vi "Simulate3DOFChair.vi"(0 "array":dbl[][](array[numeric])=[[80.0, 80.0]], 1 "L_seat":dbl=40.0, 2 "L_back":dbl=40.0, 5 "origin":cluster{"x":i16, "y":i16}, 7 "Reflection":cluster{"x":i16, "y":i16}={"x"=1, "y"=1}, 9 "L1":dbl=80.0, 11 "L2":dbl=80.0, 12 "Empty picture":picture) -> (4 "2D Picture 2":picture, 6 "point to IK":cluster{dbl, dbl})   [LabVIEW 2024]
panel:
  out "theta3":dbl(knob)=-96.67737485561672 scale=-90.0..90.0
  out "end eff coords":cluster{"x2":dbl, "y2":dbl}={"x2"=70.00000000000001, "y2"=90.0}
  out "Arm 1 coords":cluster{"x":dbl, "y":dbl}={"x"=79.30228332368782, "y"=10.542668526020577}
  in  "Empty Array 2":dbl[][](array[numeric])
  out "Drawn Coords":dbl[][](array[numeric])=[[70.00000000000001, 90.0]]
  out "angle 2":dbl=52.125016348901795
  out "mag 2":dbl=114.01754250991381
  out "end effector":cluster{dbl, dbl}={70.00000000000001, 90.0} caption="end effector 2" {"?" format="%.1f"; "?" format="%#.1f"}
  out "theta 2":dbl(knob)=89.10471701342988 scale=-90.0..90.0
  out "theta 1":dbl(knob)=7.572657842186857 scale=-90.0..90.0
  # "mm"
  # "mm"
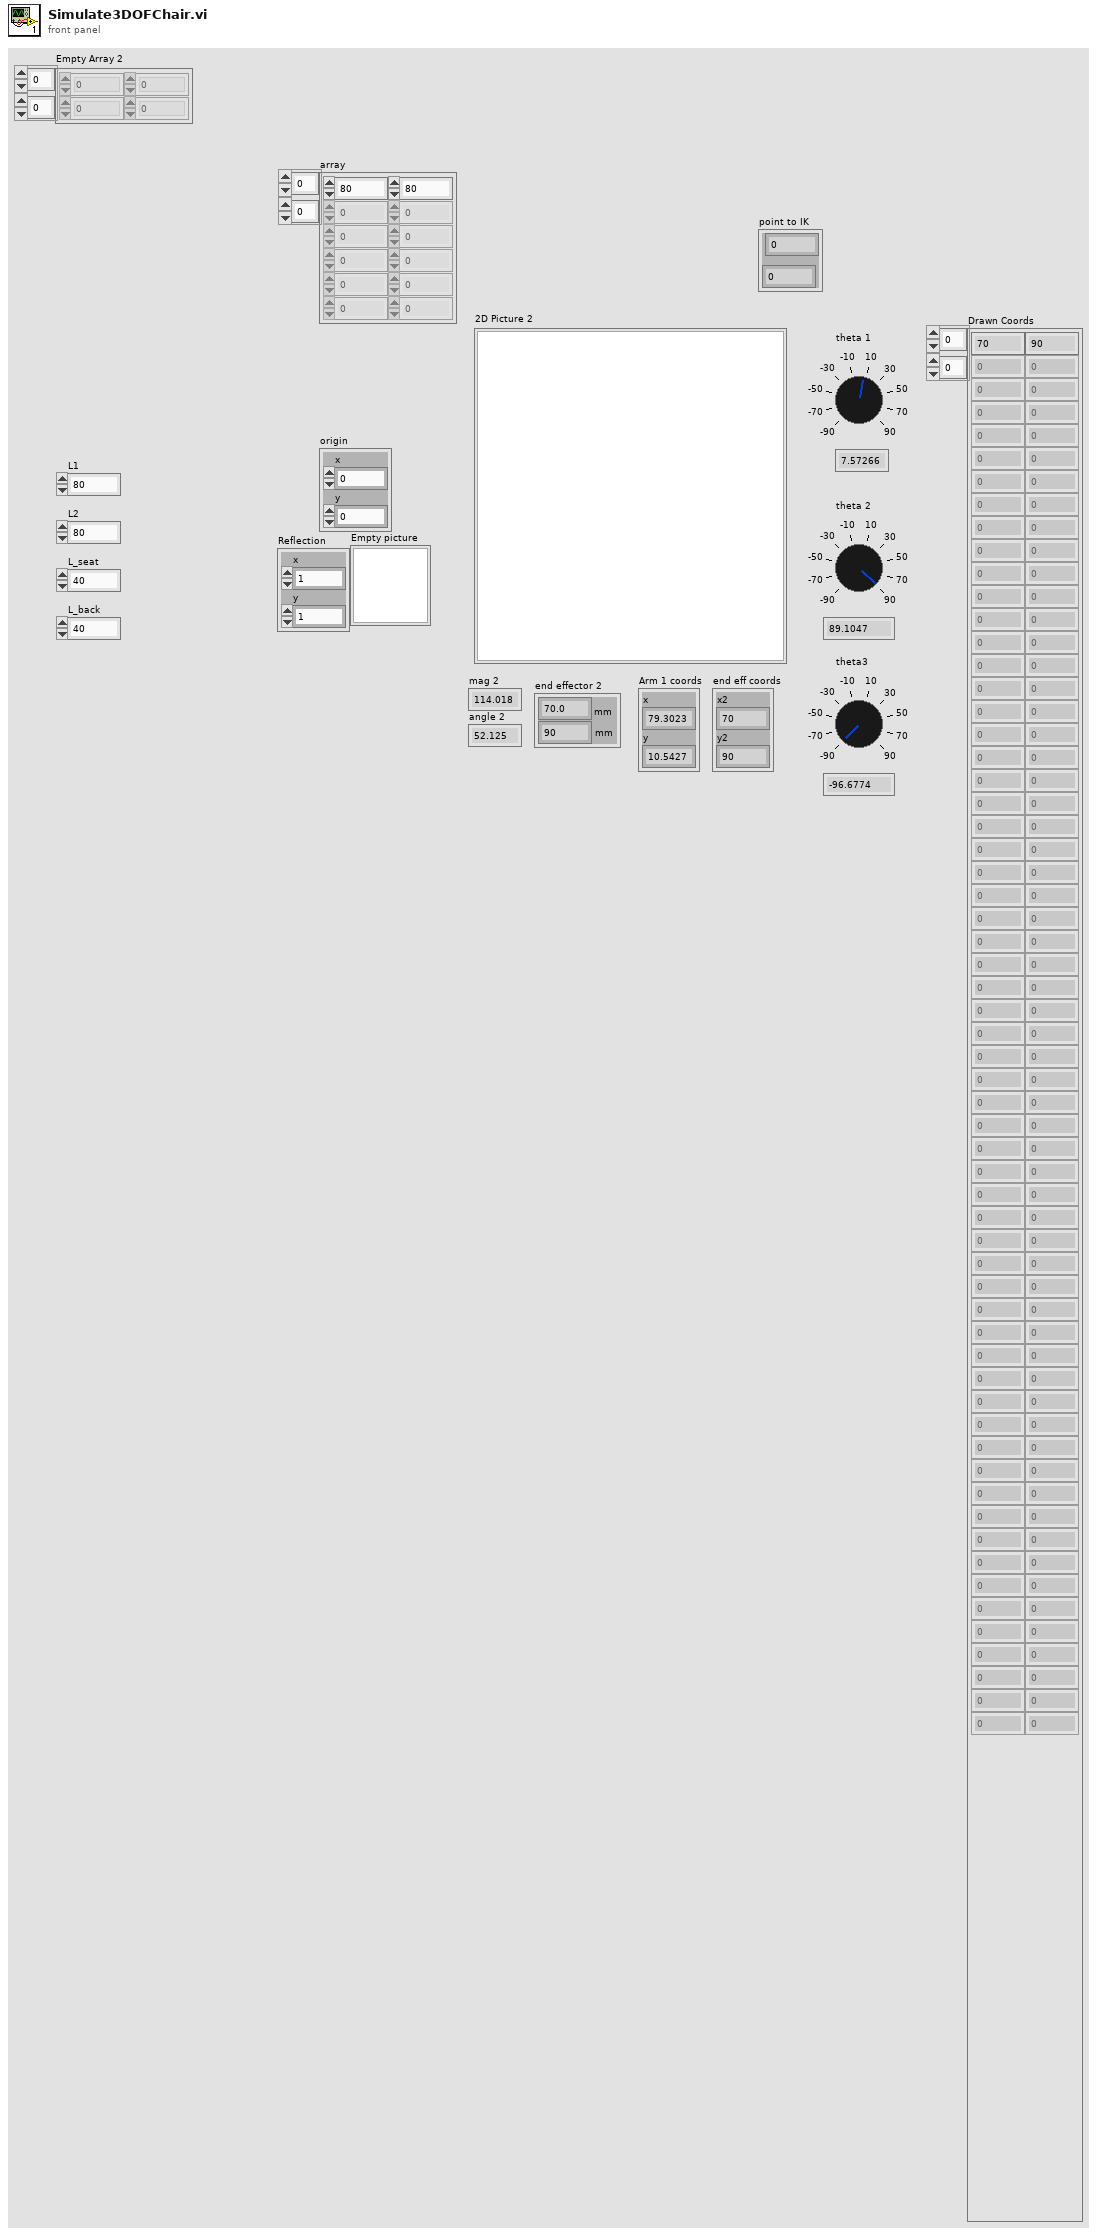
[diagram p1: front panel]
types:
  T1 = cluster{"Width":u16, "Style":enum32{"Solid", "Dash", "Dot", "DashDot", "DashDotDot"}}
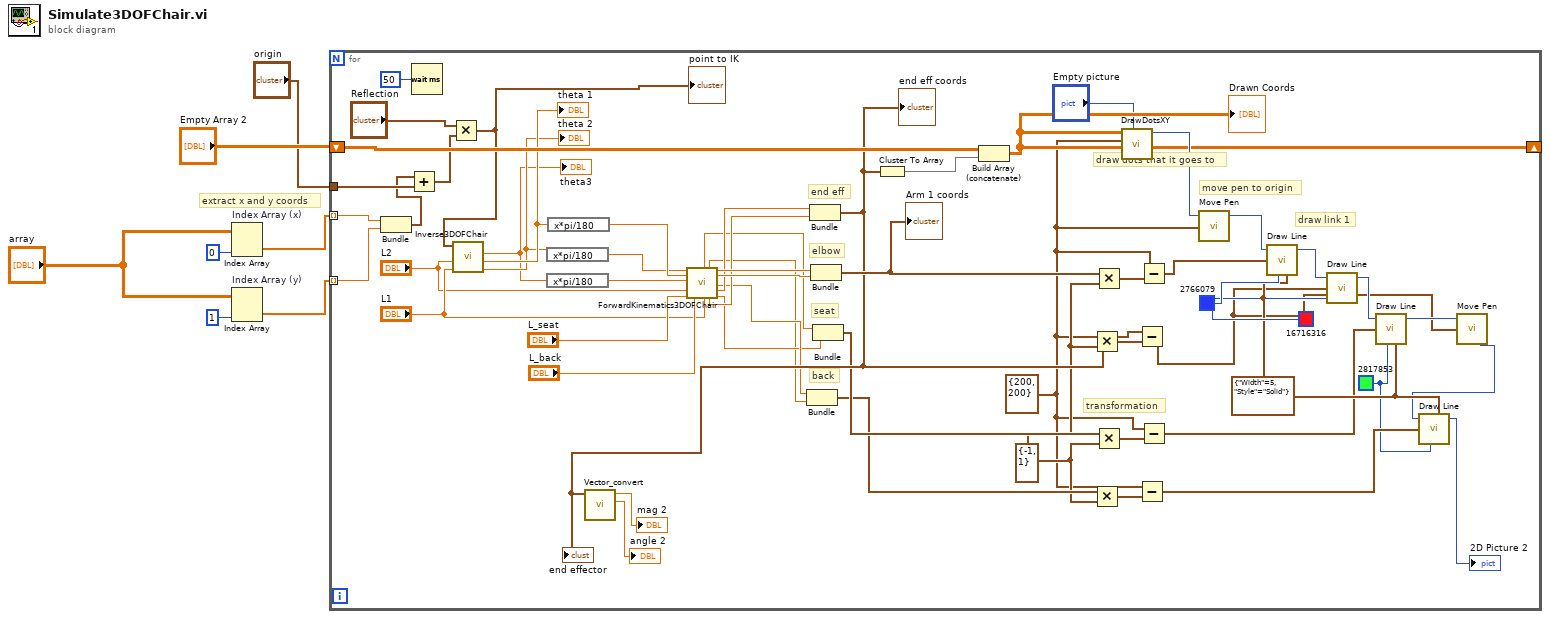
[diagram p0: block diagram]
diagram:
  # "extract x and y coords"
  n1 = Index Array "Index Array (x)"(array="array", index (col)=0 ("index (row)")) -> (element=w4:dbl[])  [unwired: 1 in]
  n2 = Index Array "Index Array (y)"(array="array", index (col)=1 ("index (row)")) -> (element=w5:dbl[])  [unwired: 1 in]
  n3 = for {
    tunnel: w4 -> [w50] mode=indexing
    tunnel: w5 -> [w49] mode=indexing
    shift-right: [w36] -> _
    shift-left: "Empty Array 2" -> [w58]
    tunnel: "origin" -> [w13]
    w24 = u32 2817853 ("color(black)")
    w27 = cluster{"x":i16, "y":i16} {"x"=-1, "y"=1} ("new position")
    w30 = T1 {"Width"=5, "Style"=enum."Solid"} ("pen")
    w26 = cluster{"x":i16, "y":i16} {"x"=200, "y"=200} ("new position")
    # "draw link 1"
    # "move pen to origin"
    # "draw dots that it goes to"
    # "back"
    # "seat"
    # "transformation"
    # "end eff"
    # "elbow"
    n4 = Bundle("y (mm)"=w50, "y (mm)"=w49) -> (w12:cluster{"y (mm)":dbl, "y (mm)":dbl})  [unwired: 1 in]
    n5 = Add(x=w12, y=w13) -> (x+y=w10:cluster{dbl, dbl})
    n6 = Wait (ms)(milliseconds to wait=u32 50) -> ()  [unwired: 1 out]
    n7 = Multiply(x="Reflection", y=w10) -> (x*y=w9:cluster{dbl, dbl})
    "point to IK" <- w9
    n8 = call "Inverse3DOFChair.vi"("L 2"="L1", "L 1"="L2", "end effector"=w9) -> ("theta2"=w17:dbl, "theta1"=w19:dbl, "theta3"=w15:dbl)  [unwired: 6 in]
    "theta 1" <- w19
    "theta 2" <- w17
    "theta3" <- w15
    n9 = expression code="x*pi/180"(w17) -> (w16:dbl)
    n10 = expression code="x*pi/180"(w15) -> (w14:dbl)
    n11 = expression code="x*pi/180"(w19) -> (w18:dbl)
    n12 = call "ForwardKinematics3DOFChair.vi"("theta2"=w16, "theta1"=w18, "L2"="L2", "seat"="L_seat", "theta3"=w14, "back"="L_back", "L1"="L1") -> ("x3"=w38:dbl, "y4"=w37:dbl, "y2"=w45:dbl, "x1"=w48:dbl, "y1"=w47:dbl, "x4"=w40:dbl, "x2"=w46:dbl, "y3"=w39:dbl)  [unwired: 5 in]
    n13 = Bundle("x4"=w40, "y4"=w37) -> (w28:cluster{"x4":dbl, "y4":dbl})  [unwired: 1 in]
    n14 = Bundle("x2"=w46, "y2"=w45) -> (w51:cluster{"x2":dbl, "y2":dbl})  [unwired: 1 in]
    "end effector" <- w51
    "end eff coords" <- w51
    n15 = call "Vector_convert.vi"("x,y"=w51) -> ("angle"=→"angle 2":dbl, "mag"=→"mag 2":dbl)  [unwired: 9 in]
    n16 = Bundle("x1"=w48, "y1"=w47) -> (w53:cluster{"x1":dbl, "y1":dbl})  [unwired: 1 in]
    "Arm 1 coords" <- w53
    n17 = Bundle("x3"=w38, "y3"=w39) -> (w32:cluster{"x3":dbl, "y3":dbl})  [unwired: 1 in]
    n18 = Cluster To Array(cluster=w51) -> (array=w59:dbl[])
    n19 = Build Array (concatenate)(w58, w59) -> (w36:dbl[][])
    "Drawn Coords" <- w36
    n20 = Multiply(x=w51, y=w27) -> (x*y=w55:cluster{dbl, dbl})
    n21 = Multiply(x=w28, y=w27) -> (x*y=w29:cluster{dbl, dbl})
    n22 = Multiply(x=w53, y=w27) -> (x*y=w54:cluster{dbl, dbl})
    n23 = Multiply(x=w32, y=w27) -> (x*y=w33:cluster{dbl, dbl})
    n24 = call "DrawDotsXY.vi"("Empty picture"="Empty picture", "new position"=w26, "Array"=w36) -> ("2D picture"=w60:picture)  [unwired: 8 in]
    n25 = Subtract(x=w26, y=w55) -> (x-y=w20:cluster{dbl, dbl})
    n26 = Subtract(x=w26, y=w29) -> (x-y=w25:cluster{dbl, dbl})
    n27 = Subtract(x=w26, y=w54) -> (x-y=w52:cluster{dbl, dbl})
    n28 = Subtract(x=w26, y=w33) -> (x-y=w21:cluster{dbl, dbl})
    n29 = call <vilib>:"Move Pen.vi"("new position"=w26, "picture"=w60) -> ("new picture"=w64:picture)  [unwired: 3 in]
    n30 = call <vilib>:"Draw Line.vi"("picture"=w64, "end point"=w52, "color(black)"=u32 2766079, "pen"=w30) -> ("new picture"=w63:picture)  [unwired: 5 in]
    n31 = call <vilib>:"Draw Line.vi"("picture"=w63, "end point"=w20, "color(black)"=u32 16716316, "pen"=w30) -> ("new picture"=w34:picture)  [unwired: 5 in]
    n32 = call <vilib>:"Draw Line.vi"("picture"=w34, "end point"=w21, "color(black)"=w24, "pen"=w30) -> ("new picture"=w23:picture)  [unwired: 5 in]
    n33 = call <vilib>:"Move Pen.vi"("new position"=w20, "picture"=w23) -> ("new picture"=w22:picture)  [unwired: 3 in]
    n34 = call <vilib>:"Draw Line.vi"("picture"=w22, "end point"=w25, "color(black)"=w24, "pen"=w30) -> ("new picture"=→"2D Picture 2":picture)  [unwired: 5 in]
  }
